vi "Queue ByteArray.vi"(8 "error in":errorcluster, 10 "bytes":u8[](array[numeric]) format="%02x", 11 "Buffer":refnum<data-value>) -> (0 "error out":errorcluster, 2 "overflow":u8[](array[numeric]) format="%02x", 3 "Buffer":refnum<data-value>)   [LabVIEW 2013, in "CircularBuffer.lvlib" / "ByteFIFO.lvclass"]
doc: "This VI allows to input an array into the buffer. The location in the buffer is updated automatically.\n\nIf the input array is larger than the buffer then just take last elements of the input array and save them in the buffer. Also give a warning that this happened."
uses:
  ByteFIFO.lvclass
  VariantBuffer/VariantBuffer.lvclass
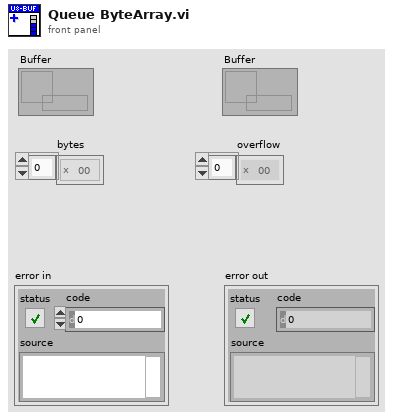
[diagram p1: front panel]
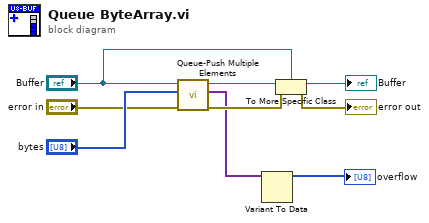
[diagram p0: block diagram]
diagram:
  n1 = call "Queue-Push Multiple Elements.vi"("error in"="error in", "elements"="bytes", "Buffer in"="Buffer") -> ("error out"=w4:errorcluster, "overflow"=w2:variant[], "Buffer"=w7:refnum<data-value>)  [unwired: 6 in]
  n2 = Variant To Data(Variant=w2) -> (data=→"overflow":u8[])  [unwired: 2 in, 1 out]
  n3 = To More Specific Class(target class="Buffer", reference=w7, error in=w4) -> (specific class reference=→"Buffer":refnum<data-value>, error out=→"error out":errorcluster)
